vi "multiColor Graph and XY Graph.vi"() -> ()   [LabVIEW 2012]
uses:
  <vilib>/Analysis/1siggen.llb/Ramp Pattern by Samples.vi
  <vilib>/measure/NI_MABase.lvlib
  <vilib>/Analysis/NI_AALBase.lvlib
panel:
  out "多颜色波形曲线":waveform(dbl)[](graph)
  out "多颜色圆形":cluster{cdb[]}[](graph)
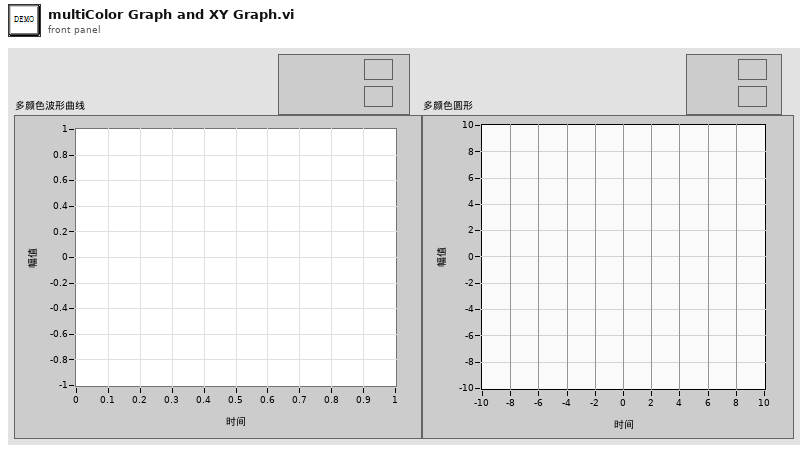
[diagram p1: front panel]
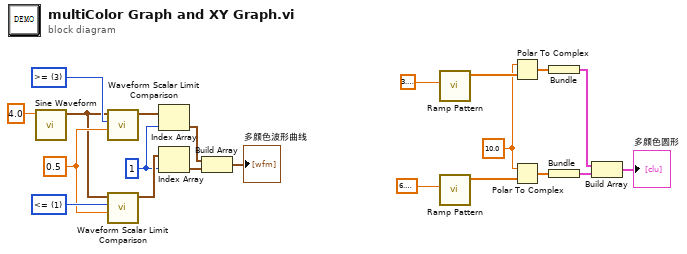
[diagram p0: block diagram]
diagram:
  w9 = 10.0
  w18 = u16 1 items=["<", "<=", ">", ">="] ("compare condition")
  w16 = 1 ("索引")
  w2 = 0.5 ("limit")
  w20 = u16 3 items=["<", "<=", ">", ">="] ("compare condition")
  n1 = call <vilib>:"Sine Waveform.vi"("frequency"=4.0) -> ("signal out"=w1:waveform(dbl))  [unwired: 9 in, 1 out]
  n2 = call <vilib>:"Waveform Scalar Limit Comparison.vi"("limit"=w2, "compare condition"=w20, "data"=w1) -> ("output waveforms"=w19:waveform(dbl)[])  [unwired: 6 in, 2 out]
  n3 = call <vilib>:"Waveform Scalar Limit Comparison.vi"("limit"=w2, "compare condition"=w18, "data"=w1) -> ("output waveforms"=w17:waveform(dbl)[])  [unwired: 6 in, 2 out]
  n4 = Index Array(array=w19, index=w16) -> (element=w15:waveform(dbl))
  n5 = Index Array(array=w17, index=w16) -> (element=w14:waveform(dbl))
  n6 = Build Array(w15, w14) -> (→"多颜色波形曲线":waveform(dbl)[])
  n7 = call-poly <vilib>:"Ramp Pattern.vi"("end"=3.141592653589793) -> ("Ramp Pattern"=w10:dbl[])  [unwired: 9 in, 1 out]
  n8 = call-poly <vilib>:"Ramp Pattern.vi"("end"=6.283185307179586) -> ("Ramp Pattern"=w11:dbl[])  [unwired: 9 in, 1 out]
  n9 = Polar To Complex(1:w10, 2:w9) -> (0:w4:cdb[])
  n10 = Polar To Complex(1:w11, 2:w9) -> (0:w8:cdb[])
  n11 = Bundle(w4) -> (w6:cluster{cdb[]})  [unwired: 1 in]
  n12 = Bundle(w8) -> (w5:cluster{cdb[]})  [unwired: 1 in]
  n13 = Build Array(w6, w5) -> (→"多颜色圆形":cluster{cdb[]}[])
